vi "New Process (Multiplot).vi"(8 "error in (no error)":errorcluster, 9 "Multiplot inputs":T1, 10 "Init options":T2={"UI visible?"=TRUE, "Update rate (ms)"=250, "visible sidebar?"=TRUE, "time to plot (init)"=600.0, "time to plot (max)"=inf, "config file start path"=path ""} {"time to plot (init)" format="%<%H:%M:%S>t"}, 11 "BluePlotHandle in":refnum<class "BluePlotHandle.lvclass">) -> (0 "error out":errorcluster, 2 "VI ref":refnum<vi>, 3 "BluePlotHandle out":refnum<class "BluePlotHandle.lvclass">)   [LabVIEW 2021, in "BluePlot.lvlib" / "BluePlotHandle.lvclass"]
doc: "This will launch a new asynchronous plot instance.\n\n<B>BluePlotHandle in\n</B>This needs to be a user-created object which has dynamic dispatch overrides for satisfying the framework of the package.\n\n<B>Init options</B>\nOptional arguments for affecting the bootup behavior of the plot instance.\nUI Visibile --> Is the UI visible? If no, then the plots are not updated.\nUpdate rate (ms) --> refresh rate of the plots\nvisible sidebar? --> Is the sidebar displaing channel names visible?\ntime to plot (init) --> initial value for the time-to-plot control\ntime to plot (max) --> max allowed entry value for the time-to-plot control\n\n<B>VI ref</B>\nThis output is a reference to the launched plot instance.\nYou are able to insert this into a subpanel, or just open the front panel directly."
uses:
  BluePlotHandle.lvclass
  SubVIs/Init Options.ctl
  TypeDefs/BlueMultiPlot Inputs.ctl
  TypeDefs/plot handle queue data.ctl
  TypeDefs/Plot QSM action.ctl
  BluePlotHandle.lvclass/BluePlotHandle.ctl
  BluePlot Main.vi
  BluePlot.lvlib
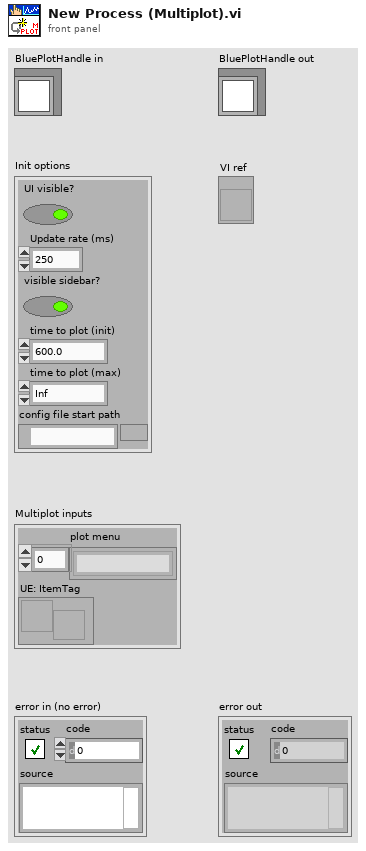
[diagram p1: front panel]
types:
  T1 = typedef "BluePlot.lvlib/BlueMultiPlot Inputs.ctl" = cluster{"plot menu":string[], "UE: ItemTag":refnum<user-event>}
  T2 = typedef "BluePlot.lvlib/BluePlotHandle.lvclass/Init Options.ctl" = cluster{"UI visible?":bool, "Update rate (ms)":u32, "visible sidebar?":bool, "time to plot (init)":dbl, "time to plot (max)":dbl, "config file start path":path}
  T3 = typedef "BluePlot.lvlib/Plot QSM action.ctl" = enum16{"start updating", "stop updating", "Shutdown", "Update", "Init", "Get Config", "Load Config"}
  T4 = typedef "BluePlot.lvlib/plot handle queue data.ctl" = cluster{"action":T3, "data":variant}
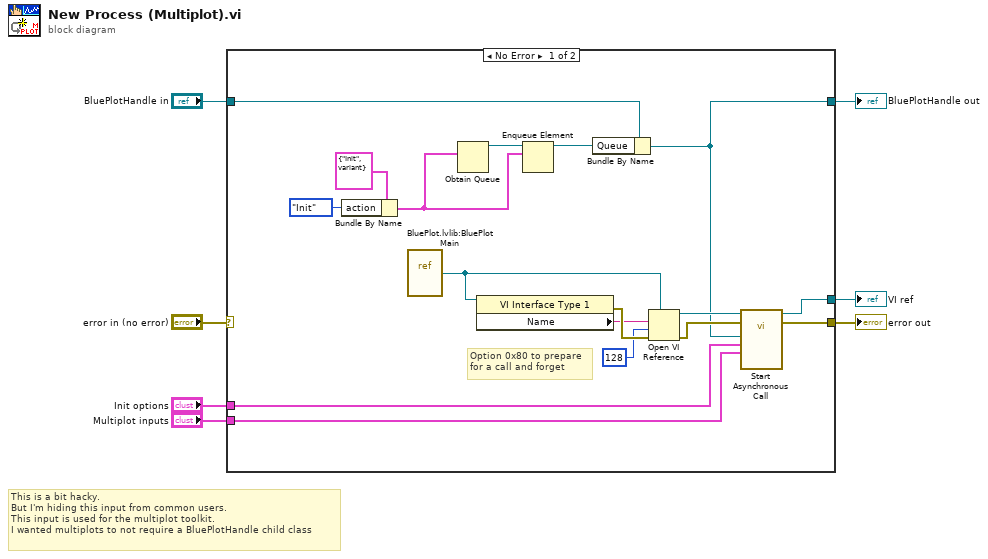
[diagram p0: block diagram]
diagram:
  # "This is a bit hacky.\nBut I'm hiding this input from common users.\nThis input is used for the multiplot toolkit.\nI wanted multiplots to not require a BluePlotHandle child class"
  n1 = case shown="No Error" "error in (no error)" {
    selector: "error in (no error)" -> [_ w26]
    tunnel: [w15 w26] -> w4
    tunnel: [w14 w25] -> w6
    tunnel: [w16 _] -> w7
    tunnel: "BluePlotHandle in" -> [w13 w25]
    tunnel: "Init options" -> [w9 _]
    tunnel: "Multiplot inputs" -> [w8 _]
    frame No Error {
      # "Option 0x80 to prepare\nfor a call and forget"
      n2 = Bundle By Name(cluster=T4 {"action"=enum."Init", "data"=variant} ("Cluster"), "action"=Plot_QSM_action."Init") -> (w10:T4)
      n3 = vi-ref "BluePlot.lvlib:BluePlot Main.vi"() -> (w21:refnum<vi>)
      n4 = Obtain Queue(element data type=w10) -> (queue out=w24:refnum<queue>)  [unwired: 4 in, 2 out]
      n5 = property class="VI Interface Type 1"(reference=w21) -> (error out=w19:errorcluster, "Name"=w18:string)  [unwired: 1 in, 1 out]
      n6 = Enqueue Element(queue=w24, element=w10) -> (queue out=w23:refnum<queue>)  [unwired: 2 in, 2 out]
      n7 = Bundle By Name(cluster=w13, "Queue"=w23) -> (w14:refnum<class "BluePlotHandle.lvclass">)
      n8 = Open VI Reference(type specifier VI Refnum (for type only)=w21, vi path=w18, options=128, error in (no error)=w19) -> (vi reference=w20:refnum<vi>, error out=w22:errorcluster)  [unwired: 2 in]
      n9 = call-by-ref "Start Asynchronous Call"(reference=w20, error in=w22, "Multiplot inputs"=w8, "Init options"=w9, "BluePlotHandle"=w14) -> (reference out=w16:refnum<vi>, error out=w15:errorcluster)  [unwired: 9 in]
    }
    frame Error {
    }
  }
  "error out" <- w4
  "BluePlotHandle out" <- w6
  "VI ref" <- w7
